vi "LINX - Servo 1 Channel.vi"() -> ()   [LabVIEW 2019]
doc: "This example demonstrates how to control a servo using LINX."
uses:
  <vilib>/MakerHub/LINX/Public/Utilities/Open Serial.vi
  <vilib>/MakerHub/LINX/Public/Sensors/Motion/Servo/Servo Open One Channel.vi
  <vilib>/MakerHub/LINX/Public/Sensors/Motion/Servo/Servo Set Pulse Width One Channel.vi
  <vilib>/MakerHub/LINX/Public/Sensors/Motion/Servo/Servo Close One Channel.vi
  <vilib>/MakerHub/LINX/LMH-LINX.lvlib
  <vilib>/MakerHub/LINX/Public/Sensors/Motion/Servo/Servo.lvlib
panel:
  in  "Servo Position":u16(knob)=1493 scale=500.0..2500.0
  in  "Servo Channel":u8=2
  in  "Stop Button":bool
  in  "Serial Port":refnum<visa-resource-name>
  # "Servo Example (Serial Interface)\n\nThis example demonstrates how to control a servo.\n\nInstructions\n1. Select the COM Port associated with the LINX Device.\n2. Select the Servo Channel connected to the servo to control.\n3. Click the Run Arrow.\n4. Adjust the dial to control the digital pulse width sent to the servo.  The pulse \n    width determines the servo position.  A 1500 uS pulse is typically 90 degrees.  \n    The maximum angle will depend on the sepcific servo used."
  # "Servo Position \n(Pulse Width uS)"
  # "LINX Device Settings"
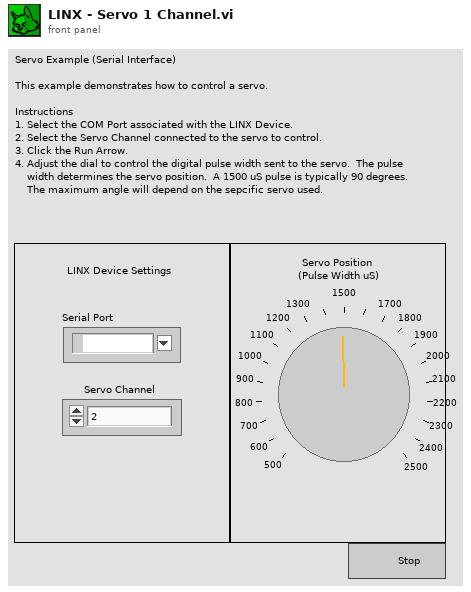
[diagram p1: front panel]
types:
  T1 = typedef "LMH-LINX.lvlib/LINX Ref.ctl" = cluster{"IO":T2, "Interface":T3, "LINX Device Config":T4}
  T2 = typedef "LMH-LINX.lvlib/Platform.ctl" = enum16{"Remote", "Local"}
  T3 = typedef "LMH-LINX.lvlib/Interface.ctl" = enum16{"Serial", "TCP"}
  T4 = typedef "LMH-LINX.lvlib/Device.lvlib/LINX Device Config.ctl" = cluster{"Interface":T3, "COM Port":refnum<visa-resource-name>, "TCP Configuration":T5, "Device Family":u8, "Device ID":u8, "Device Name":string, "TCP Ref":refnum<k5>, "Channels":T6}
  T5 = typedef "LMH-LINX.lvlib/Device.lvlib/TCP Config.ctl" = cluster{"IP Address":string, "Port":u16}
  T6 = typedef "LMH-LINX.lvlib/Channels.ctl" = cluster{"DI":u8[], "DO":u8[], "AI":u8[], "AO":u8[], "PWM":u8[], "QE":u8[], "UART":u8[], "I2C 2":u8[], "SPI":u8[], "CAN":u8[], "Servo":u8[], "AI Ref (V)":dbl, "AI Resolution (Bits)":u8, "AO Ref (V)":dbl, "AO Resolution (Bits)":u8}
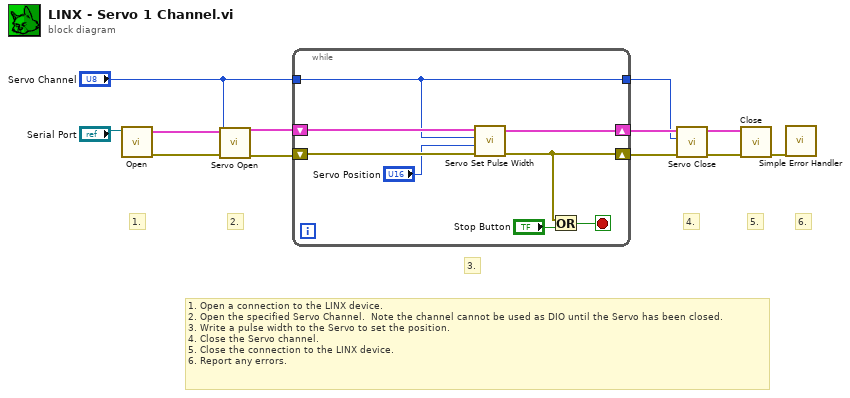
[diagram p0: block diagram]
diagram:
  # "6."
  # "1. Open a connection to the LINX device.\n2. Open the specified Servo Channel.  Note the channel cannot be used as DIO until the Servo has been closed.\n3. Write a pulse width to the Servo to set the position.\n4. Close the Servo channel.  \n5. Close the connection to the LINX device.\n6. Report any errors."
  # "5."
  # "4."
  # "3."
  # "2."
  # "1."
  n1 = call-poly <vilib>:"Open.vi"("Serial Port"="Serial Port") -> ("Error Out"=w11:errorcluster, "LINX Resource"=w10:T1)  [unwired: 8 in, 1 out]
  n2 = call-poly <vilib>:"Servo Open.vi"("Error In"=w11, "Servo Channel"="Servo Channel", "LINX Resource"=w10) -> ("Error Out"=w9:errorcluster, "LINX Resource"=w8:T1)  [unwired: 7 in]
  n3 = while {
    shift-right: [w17] -> w2
    shift-left: w9 -> [w18]
    tunnel: "Servo Channel" -> [w13]
    shift-right: [w14] -> w5
    shift-left: w8 -> [w15]
    tunnel: [w13] -> w1
    stop <- w20 stop-if-true
    n4 = call-poly <vilib>:"Servo Set Pulse Width.vi"("Error In"=w18, "Pulse Width (uS)"="Servo Position", "Servo Channel"=w13, "LINX Resource"=w15) -> ("Error Out"=w17:errorcluster, "LINX Resource"=w14:T1)  [unwired: 6 in]
    n5 = Or(x=w17, y="Stop Button") -> (x .or. y?=w20:bool)
  }
  n6 = call-poly <vilib>:"Servo Close.vi"("Error In"=w2, "Servo Channel"=w1, "LINX Resource"=w5) -> ("Error Out"=w3:errorcluster, "LINX Resource"=w4:T1)  [unwired: 7 in]
  n7 = call <vilib>:"Close.vi"("Error In"=w3, "LINX Resource"=w4) -> ("Error Out"=w6:errorcluster)  [unwired: 9 in]
  n8 = call <vilib>:"Simple Error Handler.vi"("error in (no error)"=w6) -> ()  [unwired: 4 in, 5 out]
